vi "read.vi"(8 "error in (no error)":errorcluster, 11 "Keithley2002 in":refnum<class "Keithley2002.lvclass">) -> (0 "error out":errorcluster, 2 "medicion":dbl, 3 "Keithley2002 out":refnum<class "Keithley2002.lvclass">)   [LabVIEW 2019, in "Keithley2002.lvclass"]
uses:
  Keithley2002.lvclass
panel:
  out "Reading Result":string
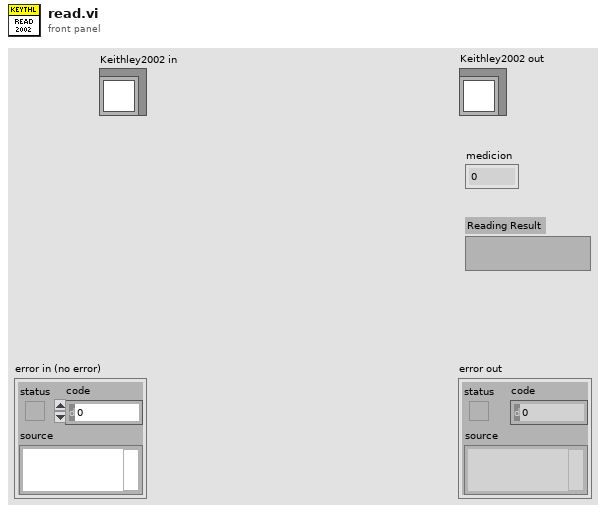
[diagram p1: front panel]
types:
  T1 = cluster{"error":bool, "code":i32, "source":string}
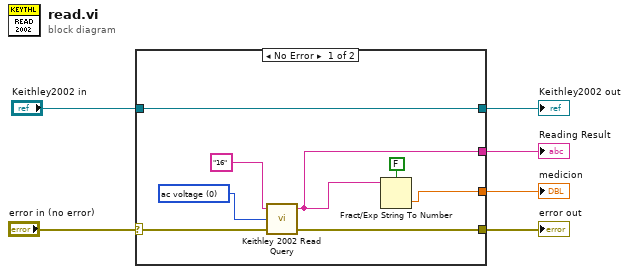
[diagram p0: block diagram]
diagram:
  n1 = case shown="No Error" "error in (no error)" {
    selector: "error in (no error)" -> [w11 w16]
    tunnel: [w10 w16] -> w5
    tunnel: [w14 w15] -> w3
    tunnel: "Keithley2002 in" -> [w14 w15]
    tunnel: [w8 _] -> w2
    tunnel: [w7 _] -> w1
    frame No Error {
      w13 = u16 0 items=["ac voltage", "dc voltage", "2-wire resistance", "4-wire resistance", "ac current", "dc current", "frequency", "temperature"] ("function (Vdc:1)")
      n2 = call <instrlib>:"Keithley 2002 Read Query.vi"("error in"=w11, "function (Vdc:1)"=w13, "GPIB Address"="16") -> ("error out"=w10:T1, "Reading Result"=w7:string)  [unwired: 1 in]
      n3 = Fract/Exp String To Number(use system decimal point (T)=FALSE, string=w7) -> (number=w8:dbl)  [unwired: 2 in, 1 out]
    }
    frame Error {
    }
  }
  "error out" <- w5
  "Keithley2002 out" <- w3
  "medicion" <- w2
  "Reading Result" <- w1
